vi "FPGA (1).vi"() -> ()   [LabVIEW 2017]
uses:
  <vilib>/rvi/Emulation/niFpgaGetClockAttributes.vi
  <vilib>/rvi/Emulation/niFpgaSctlEmulationGetInTimedLoop.vi
  <vilib>/rvi/Emulation/niFpgaEmulationReportErrorSimple.vi
  <vilib>/rvi/eio/common/nirviEmuTemplateMethod_errors.vi
  <vilib>/rvi/interface/RandomDataEmulation/niFpgaRandomDataHandleErrors.vi
  <vilib>/rvi/Emulation/niFpgaCriticalErrorInLSC.vi
  <vilib>/eio/EIONode/EIONode.xnode
  <vilib>/rvi/DataTransferAndStorage/Container/XNode/niFpgaContainer.xnode
  <vilib>/rvi/interface/RandomDataEmulation/nirviRandomDataFpgaReadWriteTemplate.vi
panel:
  out "Timed Out?":bool
  in  "Timeout":i32=5
  in  "stop":bool
  in  "Count(uSec)":u32=16
  # "Program 2f\nFPGA Front Panel"
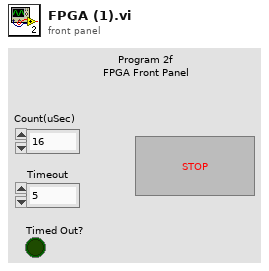
[diagram p1: front panel]
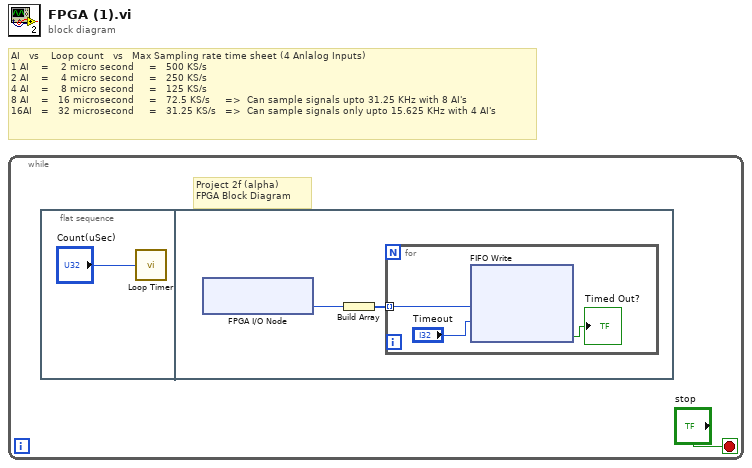
[diagram p0: block diagram]
diagram:
  # "AI   vs    Loop count   vs   Max Sampling rate time sheet (4 Anlalog Inputs)\n1 AI    =    2 micro second     =   500 KS/s\n2 AI    =    4 micro second     =   250 KS/s\n4 AI    =    8 micro second     =   125 KS/s\n8 AI    =   16 microsecond     =   72.5 KS/s     =>  Can sample signals upto 31.25 KHz with 8 AI's\n16AI   =   32 microsecond     =   31.25 KS/s   =>  Can sample signals only upto 15.625 KHz with 4 AI's"
  n1 = while {
    stop <- "stop" stop-if-true
    # "Project 2f (alpha)\nFPGA Block Diagram"
    n2 = flat-sequence {
      frame #0 {
        n3 = call "Loop Timer"("Count(uSec)"="Count(uSec)") -> ()  [unwired: 1 out]
      }
      frame #1 {
        n4 = xnode "FPGA I/O Node"() -> ("AudioIn/Left"=w4:i16)  [unwired: 1 in, 1 out]
        n5 = Build Array(w4) -> (w3:i16[])
        n6 = for {
          tunnel: w3 -> [w7] mode=indexing
          n7 = xnode ("FIFO Write")("Element"=w7, "Timeout"="Timeout") -> ("Timed Out?"=→"Timed Out?":bool)  [unwired: 1 in, 1 out]
        }
      }
    }
  }
